vi "Teleop.vi"(10 "Match Info":T1={"Autonomous Elapsed Seconds"=0.0, "TeleOp Elapsed Seconds"=0.0, "Disabled Elapsed Seconds"=0.0, "Visited Autonomous"=FALSE, "Visited TeleOp"=FALSE, "Visited Disabled"=FALSE, "Autonomous Settings"={"Autonomous Style"=enum."Independent", "VI Refnum"=refnum}}, 11 "Call Context":T2) -> ()   [LabVIEW 2013]
doc: "This VI is called for each TeleOp packet received from the DS where the robot is not disabled. It is often used to read from the joysticks and update I/O or to update setpoints for timed control loops. It should complete and return within 20 milliseconds or it may miss DS packets."
uses:
  <vilib>/Rock Robotics/WPI/DriverStation/WPI_DriverStationDerivedRobotMode.ctl
  <vilib>/Rock Robotics/WPI/DriverStation/WPI_DriverStationMatch Info.ctl
  <vilib>/Rock Robotics/WPI/Solenoid/WPI_SolenoidValue.ctl
  Robot Global Data.vi
  <vilib>/Rock Robotics/WPI/RobotDrive/WPI_RobotDriveArcadeDrive_Standard(NoSaturation).vi
  <vilib>/Rock Robotics/WPI/Solenoid/WPI_SolenoidSetEnum.vi
  <vilib>/Rock Robotics/WPI/Joystick/WPI_JoystickGetSetRefNum.vi
  <vilib>/Rock Robotics/WPI/RobotDrive/WPI_RobotDriveGetSetRefNum.vi
panel:
  out "Dog Gear T/F (Out/Engaged)":bool
  out "Intake Speed":dbl
  out "Plate T/F (Raised/Lowered)":bool
  out "Transmission T/F (Low/High)":bool
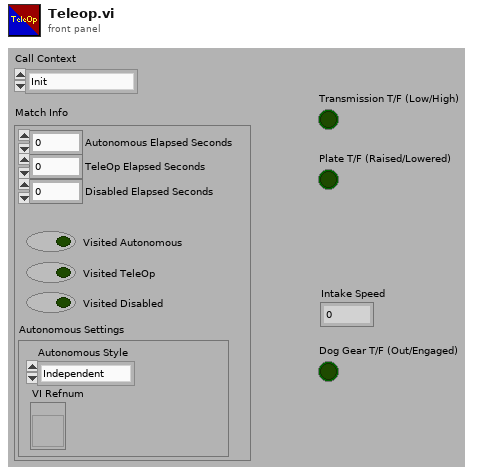
[diagram p1: front panel]
types:
  T1 = typedef "WPI_DriverStationMatch Info.ctl" = cluster{"Autonomous Elapsed Seconds":dbl, "TeleOp Elapsed Seconds":dbl, "Disabled Elapsed Seconds":dbl, "Visited Autonomous":bool, "Visited TeleOp":bool, "Visited Disabled":bool, "Autonomous Settings":cluster{"Autonomous Style":enum16{"Iterative", "Independent"}, "VI Refnum":refnum<vi>}}
  T2 = typedef "WPI_DriverStationDerivedRobotMode.ctl" = enum16{"Init", "Execute", "Stop"}
  T3 = typedef "WPI_SolenoidValue.ctl" = enum16{"Off", "On", "Forward", "Reverse"}
  T4 = typedef "WPI_JoystickDevRef.ctl" = cluster{"Device":T5}
  T5 = typedef "WPI_JoystickDeviceEnum.ctl" = enum16{"USB 1", "USB 2", "USB 3", "USB 4", "Kinect 1", "Kinect 2"}
  T6 = typedef "WPI_DigitalInputDevRef.ctl" = cluster{"DevStatus":errorcluster, "DIO Channel":T7, "Digital Module":T8}
  T7 = typedef "FPGA_DIOChannel.ctl" = enum8{"DIO 1", "DIO 2", "DIO 3", "DIO 4", "DIO 5", "DIO 6", "DIO 7", "DIO 8", "DIO 9", "DIO 10", "DIO 11", "DIO 12", "DIO 13", "DIO 14", "Invalid"}
  T8 = typedef "FPGA_TypedefDigitalModule.ctl" = enum16{"Digital Module 1", "Digital Module 2"}
  T9 = typedef "WPI_JoystickButtonState.ctl" = cluster{"Button 1":bool, "Button 2":bool, "Button 3":bool, "Button 4":bool, "Button 5":bool, "Button 6":bool, "Button 7":bool, "Button 8":bool, "Button 9":bool, "Button 10":bool, "Button 11":bool, "Button 12":bool}
  T10 = cluster{"axis 1 (x)":dbl, "axis 2 (y)":dbl, "axis 3 (throttle)":dbl, "axis 4":dbl, "axis 5":dbl, "axis 6":dbl}
  T11 = typedef "WPI_RobotDriveDevRef.ctl" = cluster{"DevStatus":errorcluster, "Motors[]":T12[], "Square Inputs":bool, "Max Output":dbl, "Isochronous":bool}
  T12 = typedef "WPI_MotorControlDeviceRef.ctl" = cluster{"DeviceStatus":errorcluster, "Type":enum16{"PWM", "CAN"}, "PWM":cluster{"Digital Module":T8, "PWM Channel":T13, "DeadBand":T14}, "CAN":cluster{"Device Number":u8, "Control Mode":T15, "Semaphore":T16, "Max Vout":dbl}, "Invert":bool, "TransformRef":T17, "InvTransformRef":T17}
  T13 = typedef "FPGA_DIOPWMChannel.ctl" = enum8{"PWM 1", "PWM 2", "PWM 3", "PWM 4", "PWM 5", "PWM 6", "PWM 7", "PWM 8", "PWM 9", "PWM 10", "Invalid"}
  T14 = typedef "WPI_PWMDeadband.ctl" = cluster{"Name":string, "maxPositivePwm":i32, "minPositivePwm":i32, "centerPwm":i32, "maxNegativePwm":i32, "minNegativePwm":i32, "angularRange":u16}
  T15 = typedef "WPI_CANJaguar_ControlMode.ctl" = enum8{"Percent VBus", "Current", "Speed", "Position", "Voltage"}
  T16 = typedef "Semaphore RefNum" = refnum<k1>
  T17 = typedef "WPI_PWMTransform_ConPane.ctl" = refnum<vi>
  T18 = typedef "WPI_SolenoidDevRef.ctl" = cluster{"DevStatus":errorcluster, "Solenoid Module":T19, "Forward Solenoid Channel":T20, "Reverse Solenoid Channel":T20}
  T19 = typedef "FPGA_TypedefSolenoidModule.ctl" = enum16{"Solenoid Module 1", "Solenoid Module 2"}
  T20 = typedef "WPI_SolenoidChannel.ctl" = enum8{"Solenoid 1", "Solenoid 2", "Solenoid 3", "Solenoid 4", "Solenoid 5", "Solenoid 6", "Solenoid 7", "Solenoid 8", "Invalid"}
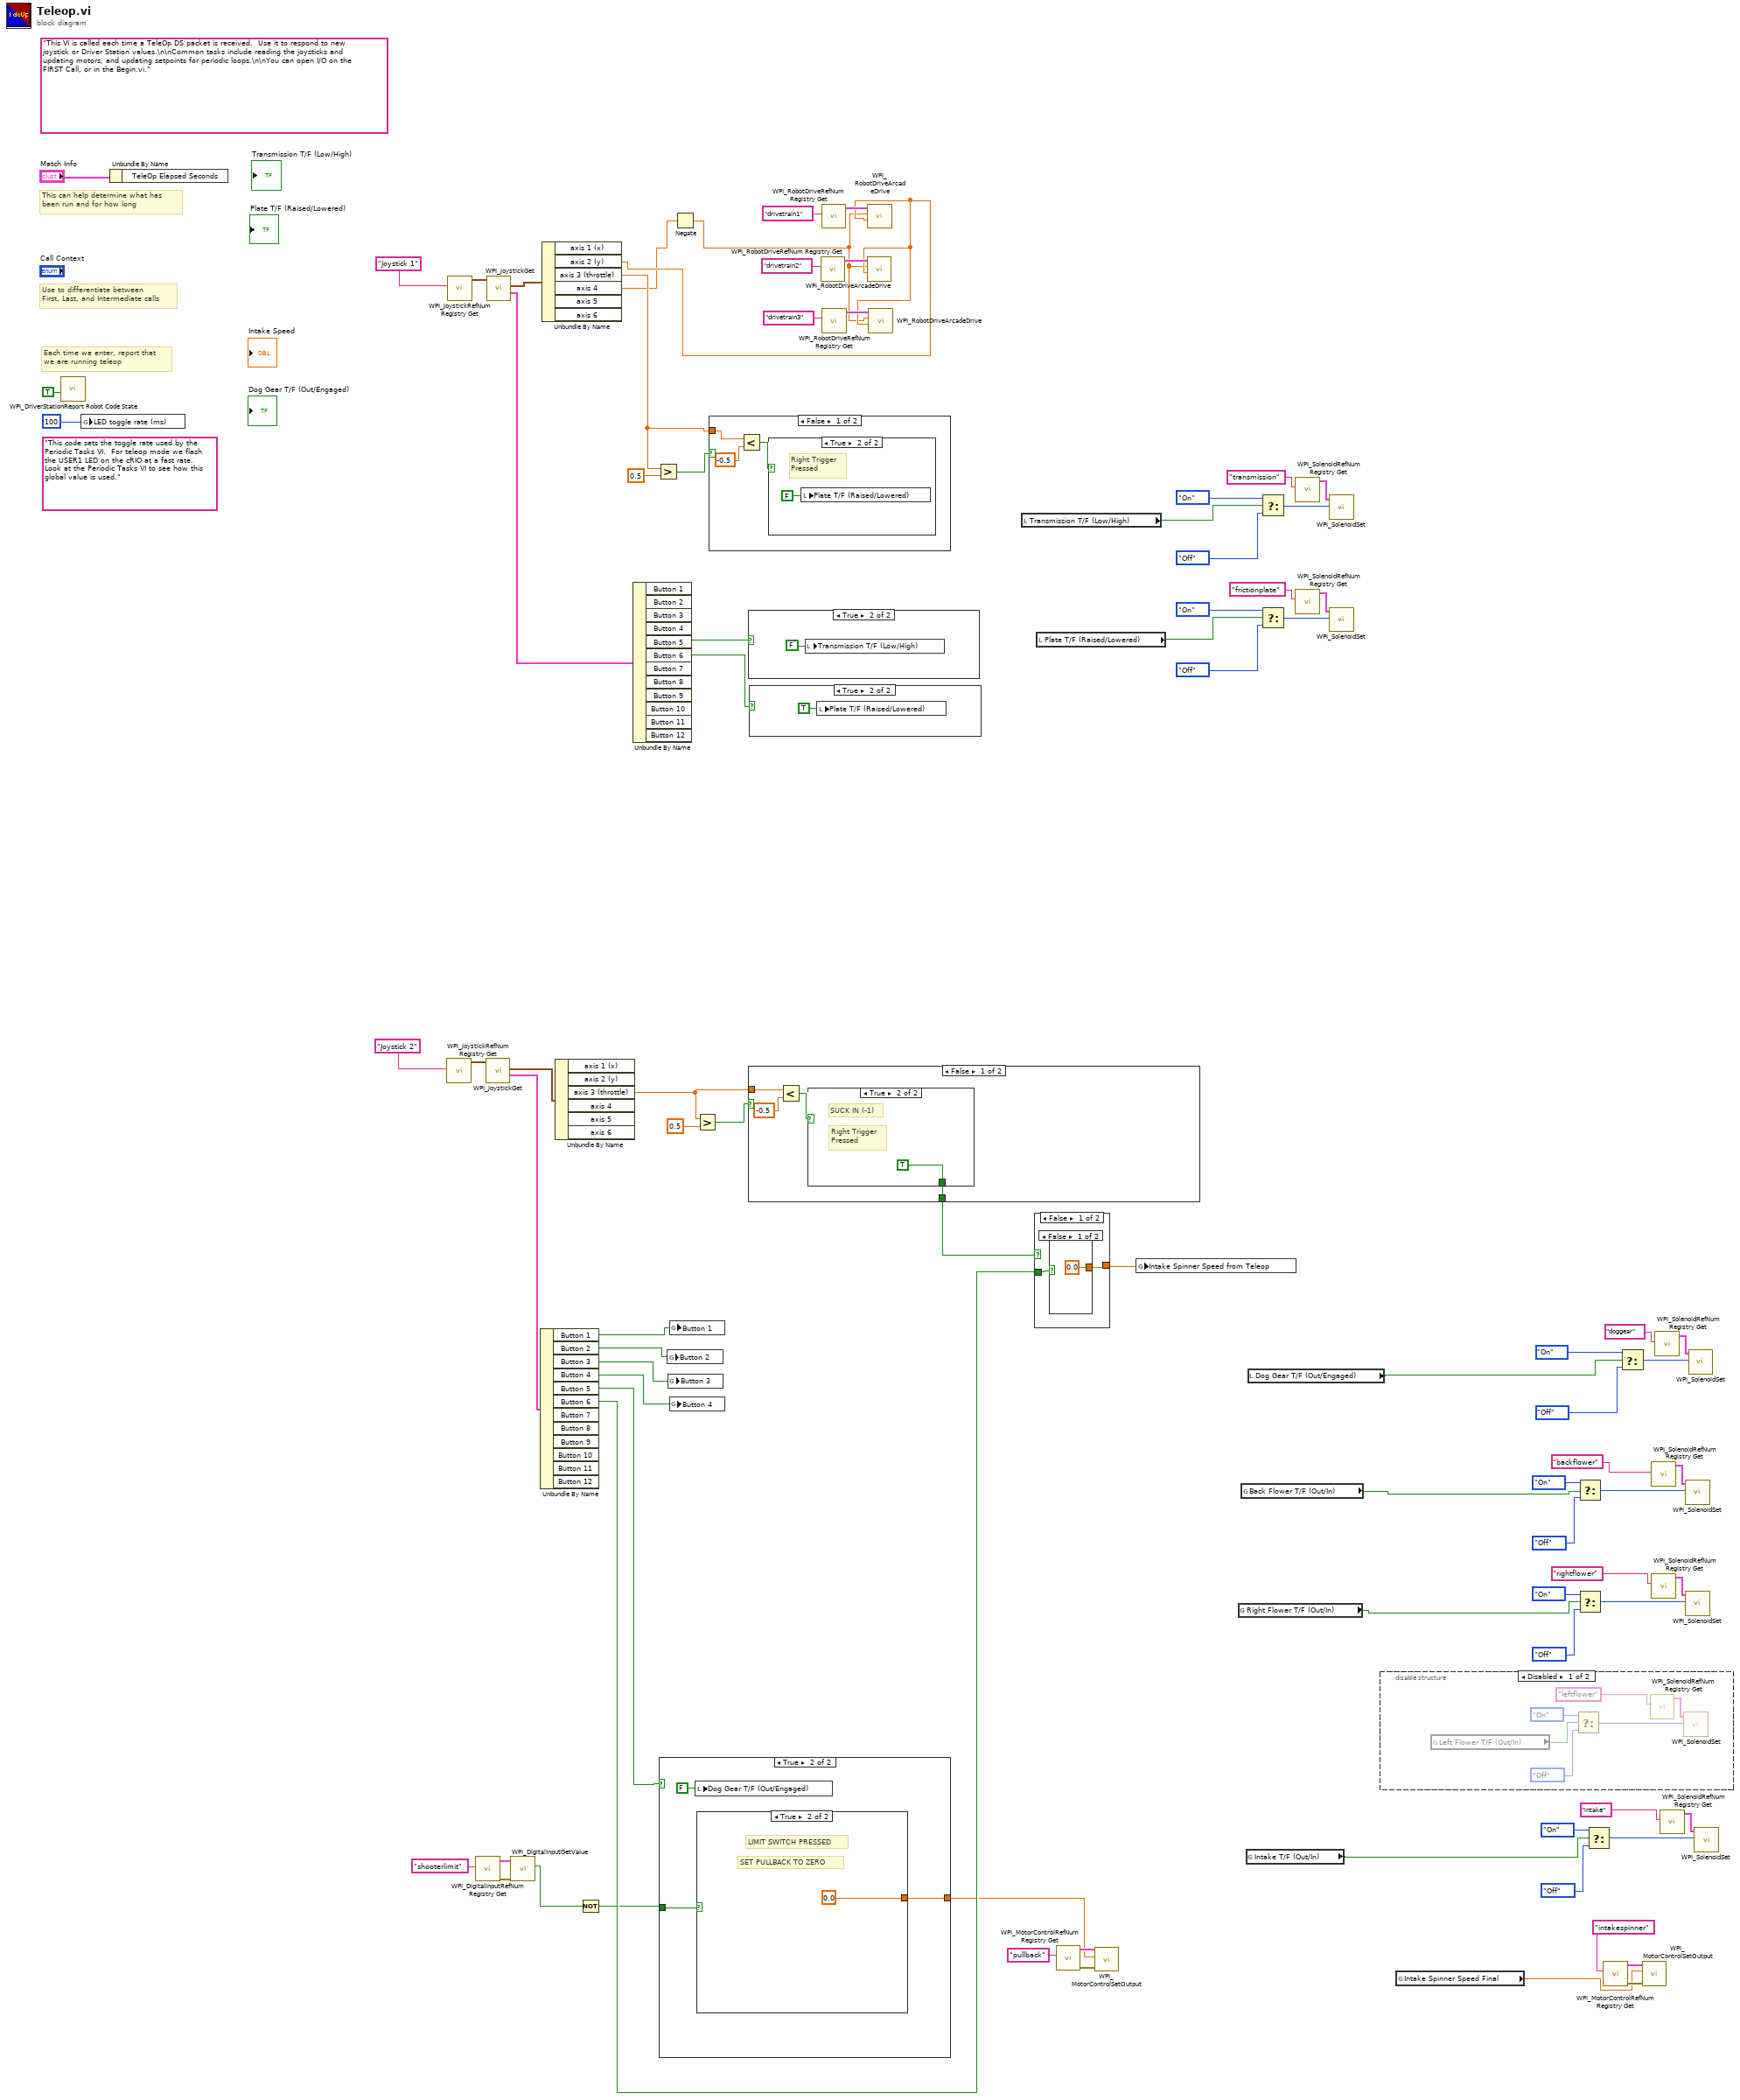
[diagram p0: block diagram]
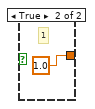
[diagram p2: hidden frame]
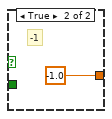
[diagram p3: hidden frame]
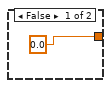
[diagram p4: hidden frame]
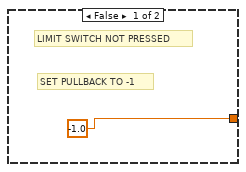
[diagram p5: hidden frame]
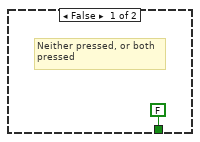
[diagram p6: hidden frame]
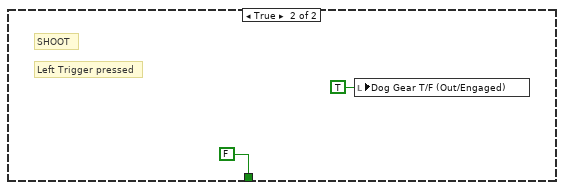
[diagram p7: hidden frame]
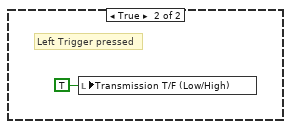
[diagram p12: hidden frame]
diagram:
  (unwired) "This code sets the toggle rate used by the Periodic Tasks VI.  For teleop mode we flash the USER1 LED on the cRIO at a fast rate.  Look at the Periodic Tasks VI to see how this global value is used."
  (unwired) "This VI is called each time a TeleOp DS packet is received.  Use it to respond to new joystick or Driver Station values.\n\nCommon tasks include reading the joysticks and updating motors, and updating setpoints for periodic loops.\n\nYou can open I/O on the FIRST Call, or in the Begin.vi."
  # "Each time we enter, report that\nwe are running teleop"
  # "Use to differentiate between\nFirst, Last, and Intermediate calls"
  # "This can help determine what has\nbeen run and for how long"
  n1 = call <vilib>:"WPI_DriverStationReport Robot Code State.vi"("TeleOp"=TRUE ("Autonomous")) -> ()  [unwired: 10 in, 1 out]
  n2 = global write "Robot Global Data.vi" "LED toggle rate (ms)"(u32 100 ("LED ms toggle rate")) -> ()
  n3 = Unbundle By Name("Match Info") -> ()  [unwired: 1 out]
  n4 = call <vilib>:"WPI_JoystickRefNum Registry Get.vi"("refnum name"="Joystick 2") -> ("JoystickDevRef"=w31:T4)  [unwired: 1 in, 9 out]
  n5 = call <vilib>:"WPI_JoystickRefNum Registry Get.vi"("refnum name"="Joystick 1") -> ("JoystickDevRef"=w81:T4)  [unwired: 1 in, 9 out]
  n6 = call <vilib>:"WPI_DigitalInputRefNum Registry Get.vi"("refnum name"="shooterlimit") -> ("error out"=w22:errorcluster, "DigitalInputDevRef"=w21:T6)  [unwired: 9 in]
  n7 = call <vilib>:"WPI_JoystickGet.vi"("JoystickDevRef"=w31) -> ("Buttons"=w30:T9, "Axes"=w29:T10)  [unwired: 1 in, 4 out]
  n8 = call <vilib>:"WPI_JoystickGet.vi"("JoystickDevRef"=w81) -> ("Buttons"=w79:T9, "Axes"=w80:T10)  [unwired: 1 in, 4 out]
  n9 = call <vilib>:"WPI_DigitalInputGetValue.vi"("error in (no error)"=w22, "DigitalInputDevRef"=w21) -> ("Value"=w10:bool)  [unwired: 7 in, 2 out]
  n10 = Unbundle By Name(w30) -> ("Button 1"=w15:bool, "Button 2"=w14:bool, "Button 3"=w13:bool, "Button 4"=w12:bool, "Button 5"=w25:bool, "Button 6"=w24:bool)  [unwired: 6 out]
  n11 = Unbundle By Name(w80) -> ("axis 2 (y)"=w35:dbl, "axis 3 (throttle)"=w70:dbl, "axis 4"=w34:dbl)  [unwired: 3 out]
  n12 = Unbundle By Name(w29) -> ("axis 3 (throttle)"=w23:dbl)  [unwired: 5 out]
  n13 = Not(x=w10) -> (.not. x?=w11:bool)
  n14 = Unbundle By Name(w79) -> ("Button 5"=w69:bool, "Button 6"=w68:bool)  [unwired: 10 out]
  n15 = Greater?(x=w70, y=0.5) -> (0:w71:bool)
  n16 = case shown="True" w25 {
    tunnel: w11 -> [_ w88]
    tunnel: [0.0 ("Output") w87] -> w16
    frame False {
    }
    frame True {
      n17 = local write "Dog Gear T/F (Out/Engaged)"(FALSE ("Dog Gear T/F (Engaged/Out)")) -> ()
      n18 = case shown="True" w88 {
        tunnel: [-1.0 ("Output") 0.0 ("Output")] -> w87
        frame False {
          # "LIMIT SWITCH NOT PRESSED"
          # "SET PULLBACK TO -1"
        }
        frame True {
          # "LIMIT SWITCH PRESSED"
          # "SET PULLBACK TO ZERO"
        }
      }
    }
  }
  n19 = global write "Robot Global Data.vi" "Button 2"(w14) -> ()
  n20 = global write "Robot Global Data.vi" "Button 3"(w13) -> ()
  n21 = global write "Robot Global Data.vi" "Button 1"(w15) -> ()
  n22 = global write "Robot Global Data.vi" "Button 4"(w12) -> ()
  n23 = Negate(x=w34) -> (-x=w33:dbl)
  n24 = Greater?(x=w23, y=0.5) -> (0:w27:bool)
  n25 = case shown="False" w71 {
    tunnel: w70 -> [w94 _]
    frame False {
      n26 = Less?(x=w94, y=-0.5) -> (x < y?=w92:bool)
      n27 = case shown="True" w92 {
        frame False {
          # "Neither pressed, or both\npressed"
        }
        frame True {
          # "Right Trigger\nPressed"
          n28 = local write "Plate T/F (Raised/Lowered)"(FALSE ("Plate T/F (Lowered/Raised)")) -> ()
        }
      }
    }
    frame True {
      # "Left Trigger pressed"
      n29 = local write "Transmission T/F (Low/High)"(TRUE ("Transmission T/F (High/Low)")) -> ()
    }
  }
  n30 = case shown="True" w69 {
    frame False {
    }
    frame True {
      n31 = local write "Transmission T/F (Low/High)"(FALSE ("Transmission T/F (High/Low)")) -> ()
    }
  }
  n32 = case shown="False" w27 {
    tunnel: [w99 FALSE] -> w26
    tunnel: w23 -> [w98 _]
    frame False {
      n33 = Less?(x=w98, y=-0.5) -> (x < y?=w100:bool)
      n34 = case shown="True" w100 {
        tunnel: [FALSE TRUE] -> w99
        frame False {
          # "Neither pressed, or both\npressed"
        }
        frame True {
          # "SUCK IN (-1)"
          # "Right Trigger\nPressed"
        }
      }
    }
    frame True {
      # "SHOOT"
      # "Left Trigger pressed"
      n35 = local write "Dog Gear T/F (Out/Engaged)"(TRUE ("Dog Gear T/F (Engaged/Out)")) -> ()
    }
  }
  n36 = case shown="True" w68 {
    frame False {
    }
    frame True {
      n37 = local write "Plate T/F (Raised/Lowered)"(TRUE ("Plate T/F (Lowered/Raised)")) -> ()
    }
  }
  n38 = call <vilib>:"WPI_RobotDriveRefNum Registry Get.vi"("refnum name"="drivetrain2") -> ("RobotDriveDevRef"=w74:T11)  [unwired: 9 in, 1 out]
  n39 = call <vilib>:"WPI_RobotDriveRefNum Registry Get.vi"("refnum name"="drivetrain1") -> ("RobotDriveDevRef"=w75:T11)  [unwired: 9 in, 1 out]
  n40 = call <vilib>:"WPI_RobotDriveRefNum Registry Get.vi"("refnum name"="drivetrain3") -> ("RobotDriveDevRef"=w73:T11)  [unwired: 9 in, 1 out]
  n41 = call-poly <vilib>:"WPI_RobotDriveArcadeDrive.vi"("Y axis value"=w35, "X axis value"=w33, "RobotDriveDevRef"=w74) -> ()  [unwired: 6 in, 3 out]
  n42 = call-poly <vilib>:"WPI_RobotDriveArcadeDrive.vi"("Y axis value"=w35, "X axis value"=w33, "RobotDriveDevRef"=w75) -> ()  [unwired: 6 in, 3 out]
  n43 = call-poly <vilib>:"WPI_RobotDriveArcadeDrive.vi"("Y axis value"=w35, "X axis value"=w33, "RobotDriveDevRef"=w73) -> ()  [unwired: 6 in, 3 out]
  n44 = local read "Transmission T/F (Low/High)"() -> (w57:bool)
  n45 = case shown="False" w26 {
    tunnel: [w107 -1.0 ("Output")] -> w5
    tunnel: w24 -> [w108 _]
    frame False {
      n46 = case shown="False" w108 {
        tunnel: [0.0 ("Output") 1.0 ("Output")] -> w107
        frame False {
        }
        frame True {
          # "1"
        }
      }
    }
    frame True {
      # "-1"
    }
  }
  n47 = local read "Plate T/F (Raised/Lowered)"() -> (w56:bool)
  n48 = call <vilib>:"WPI_MotorControlRefNum Registry Get.vi"("refnum name"="pullback") -> ("error out"=w19:errorcluster, "MotorControlDevRef"=w18:T12)  [unwired: 9 in]
  n49 = call <vilib>:"WPI_MotorControlSetOutput.vi"("error in (no error)"=w19, "Output"=w16, "MotorControlDevRef"=w18) -> ()  [unwired: 6 in, 3 out]
  n50 = global write "Robot Global Data.vi" "Intake Spinner Speed from Teleop"(w5) -> ()
  n51 = global read "Robot Global Data.vi" "Right Flower T/F (Out/In)"() -> (w6:bool)
  n52 = global read "Robot Global Data.vi" "Back Flower T/F (Out/In)"() -> (w8:bool)
  n53 = global read "Robot Global Data.vi" "Intake T/F (Out/In)"() -> (w7:bool)
  n54 = local read "Dog Gear T/F (Out/Engaged)"() -> (w9:bool)
  n55 = Select(t=WPI_SolenoidValue."On" ("Value"), s=w57, f=WPI_SolenoidValue."Off" ("Value")) -> (s? t:f=w65:T3)
  n56 = Select(t=WPI_SolenoidValue."On" ("Value"), s=w56, f=WPI_SolenoidValue."Off" ("Value")) -> (s? t:f=w60:T3)
  n57 = call <vilib>:"WPI_SolenoidRefNum Registry Get.vi"("refnum name"="transmission") -> ("SolenoidDevRef"=w63:T18)  [unwired: 9 in, 1 out]
  n58 = call <vilib>:"WPI_SolenoidRefNum Registry Get.vi"("refnum name"="frictionplate") -> ("SolenoidDevRef"=w58:T18)  [unwired: 9 in, 1 out]
  n59 = call-poly <vilib>:"WPI_SolenoidSet.vi"("Value"=w65, "SolenoidDevRef"=w63) -> ()  [unwired: 8 in, 2 out]
  n60 = call-poly <vilib>:"WPI_SolenoidSet.vi"("Value"=w60, "SolenoidDevRef"=w58) -> ()  [unwired: 8 in, 2 out]
  n61 = disable-structure shown="Disabled" {
    frame Disabled {
      n62 = global read "Robot Global Data.vi" "Left Flower T/F (Out/In)"() -> (w112:bool)
      n63 = Select(t=WPI_SolenoidValue."On" ("Value"), s=w112, f=WPI_SolenoidValue."Off" ("Value")) -> (s? t:f=w115:T3)
      n64 = call <vilib>:"WPI_SolenoidRefNum Registry Get.vi"("refnum name"="leftflower") -> ("SolenoidDevRef"=w113:T18)  [unwired: 9 in, 1 out]
      n65 = call-poly <vilib>:"WPI_SolenoidSet.vi"("Value"=w115, "SolenoidDevRef"=w113) -> ()  [unwired: 8 in, 2 out]
    }
    frame Enabled {
    }
  }
  n66 = global read "Robot Global Data.vi" "Intake Spinner Speed Final"() -> (w1:dbl)
  n67 = Select(t=WPI_SolenoidValue."On" ("Value"), s=w8, f=WPI_SolenoidValue."Off" ("Value")) -> (s? t:f=w38:T3)
  n68 = Select(t=WPI_SolenoidValue."On" ("Value"), s=w6, f=WPI_SolenoidValue."Off" ("Value")) -> (s? t:f=w48:T3)
  n69 = Select(t=WPI_SolenoidValue."On" ("Value"), s=w7, f=WPI_SolenoidValue."Off" ("Value")) -> (s? t:f=w43:T3)
  n70 = call <vilib>:"WPI_MotorControlRefNum Registry Get.vi"("refnum name"="intakespinner") -> ("error out"=w4:errorcluster, "MotorControlDevRef"=w3:T12)  [unwired: 9 in]
  n71 = Select(t=WPI_SolenoidValue."On" ("Value"), s=w9, f=WPI_SolenoidValue."Off" ("Value")) -> (s? t:f=w53:T3)
  n72 = call <vilib>:"WPI_MotorControlSetOutput.vi"("error in (no error)"=w4, "Output"=w1, "MotorControlDevRef"=w3) -> ()  [unwired: 6 in, 3 out]
  n73 = call <vilib>:"WPI_SolenoidRefNum Registry Get.vi"("refnum name"="backflower") -> ("SolenoidDevRef"=w36:T18)  [unwired: 9 in, 1 out]
  n74 = call <vilib>:"WPI_SolenoidRefNum Registry Get.vi"("refnum name"="rightflower") -> ("SolenoidDevRef"=w46:T18)  [unwired: 9 in, 1 out]
  n75 = call <vilib>:"WPI_SolenoidRefNum Registry Get.vi"("refnum name"="doggear") -> ("SolenoidDevRef"=w51:T18)  [unwired: 9 in, 1 out]
  n76 = call <vilib>:"WPI_SolenoidRefNum Registry Get.vi"("refnum name"="intake") -> ("SolenoidDevRef"=w41:T18)  [unwired: 9 in, 1 out]
  n77 = call-poly <vilib>:"WPI_SolenoidSet.vi"("Value"=w38, "SolenoidDevRef"=w36) -> ()  [unwired: 8 in, 2 out]
  n78 = call-poly <vilib>:"WPI_SolenoidSet.vi"("Value"=w48, "SolenoidDevRef"=w46) -> ()  [unwired: 8 in, 2 out]
  n79 = call-poly <vilib>:"WPI_SolenoidSet.vi"("Value"=w53, "SolenoidDevRef"=w51) -> ()  [unwired: 8 in, 2 out]
  n80 = call-poly <vilib>:"WPI_SolenoidSet.vi"("Value"=w43, "SolenoidDevRef"=w41) -> ()  [unwired: 8 in, 2 out]
